vi "Begin.vi"(8 "error in":errorcluster) -> (0 "error out":errorcluster)   [LabVIEW 2019]
doc: "Called before other user functions, this VI is expected to open initial I/O refnums, load in file data, and do all program initialization. Notice that the <B>error out</B> terminal is simply used for data flow. Wiring it to other structures or subVIs ensures that this VI runs first."
uses:
  <vilib>/Rock Robotics/WPI/DriverStation/WPI_DriverStationRobotMode2.ctl
  <vilib>/Rock Robotics/WPI/Joystick/WPI_JoystickDeviceEnum.ctl
  <vilib>/Rock Robotics/WPI/ThirdParty/Phoenix-LabVIEW/Motor Controller/Controls/CTRE_Phoenix_MotorControl_NeutralMode.ctl
  Robot Global Data.vi
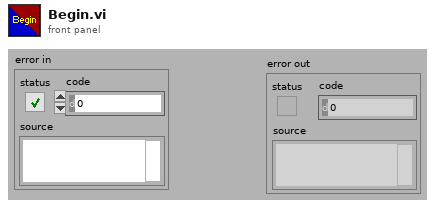
[diagram p1: front panel]
types:
  T1 = typedef "CTRE_Phoenix_MotorControl_NeutralMode.ctl" = enum8{"EEPROMSetting", "Override to Coast", "Override to Brake"}
  T2 = typedef "WPI_JoystickDeviceEnum.ctl" = enum16{"USB 0", "USB 1", "USB 2", "USB 3", "USB 4", "USB 5"}
  T3 = typedef "WPI_DriverStationRobotMode2.ctl" = enum16{"Autonomous Disabled", "Autonomous Enabled", "Teleop Disabled", "Teleop Enabled", "Disconnected", "Finish", "Test Disabled", "Test Enabled", "Emergency Stopped"}
  T4 = typedef "WPI_JoystickDevRef.ctl" = cluster{"Device":T2}
  T5 = typedef "WPI_MotorControlDeviceRef.ctl" = cluster{"DeviceStatus":errorcluster, "Type":T6, "PWM":cluster{"PWM Channel":T7, "DeadBand":T8}, "CAN":cluster{"Device Number":u8, "SetOutput VI Ref":variant, "GetOutput VI Ref":variant, "Enable VI Ref":variant, "Disable VI Ref":variant, "Data":variant}, "Invert":bool, "DIO PWM":cluster{"PWM \"Enable\" Channel":T7, "DIOChannel":T9, "PWM Rate":dbl}}
  T6 = typedef "WPI_MotorControlType.ctl" = enum16{"PWM", "CAN", "DIO PWM"}
  T7 = typedef "FPGA_DIOPWMChannel.ctl" = enum8{"PWM 0", "PWM 1", "PWM 2", "PWM 3", "PWM 4", "PWM 5", "PWM 6", "PWM 7", "PWM 8", "PWM 9", "PWM MXP 0", "PWM MXP 1", "PWM MXP 2", "PWM MXP 3", "PWM MXP 4", "PWM MXP 5", "PWM MXP 6", "PWM MXP 7", "PWM MXP 8", "PWM MXP 9", "Invalid"}
  T8 = typedef "WPI_PWMDeadband.ctl" = cluster{"Name":string, "maxPositivePwm":i32, "minPositivePwm":i32, "centerPwm":i32, "maxNegativePwm":i32, "minNegativePwm":i32, "angularRange":u16}
  T9 = typedef "FPGA_DIOChannel.ctl" = enum8{"DIO 0", "DIO 1", "DIO 2", "DIO 3", "DIO 4", "DIO 5", "DIO 6", "DIO 7", "DIO 8", "DIO 9", "DIO MXP 0", "DIO MXP 1", "DIO MXP 2", "DIO MXP 3", "DIO MXP 4", "DIO MXP 5", "DIO MXP 6", "DIO MXP 7", "DIO MXP 8", "DIO MXP 9", "DIO MXP 10", "DIO MXP 11", "DIO MXP 12", "DIO MXP 13", "DIO MXP 14", "DIO MXP 15", "SPI Port CS1", "SPI Port CS2", "SPI Port CS3", "SPI Port MISO", "SPI Port MOSI", "Invalid"}
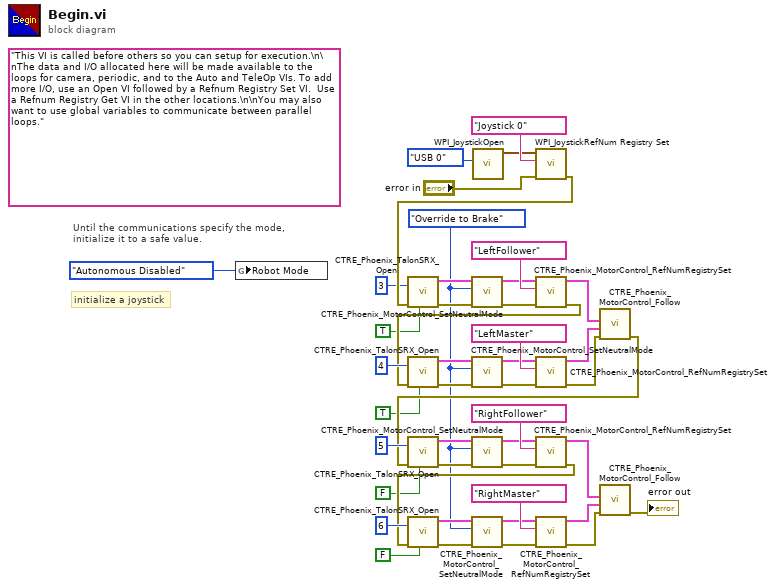
[diagram p0: block diagram]
diagram:
  w5 = CTRE_Phoenix_MotorControl_NeutralMode."Override to Brake" ("Motor Control Neutral Mode")
  (unwired) "This VI is called before others so you can setup for execution.\n\nThe data and I/O allocated here will be made available to the loops for camera, periodic, and to the Auto and TeleOp VIs. To add more I/O, use an Open VI followed by a Refnum Registry Set VI.  Use a Refnum Registry Get VI in the other locations.\n\nYou may also want to use global variables to communicate between parallel loops."
  # "initialize a joystick"
  # "Until the communications specify the mode,\ninitialize it to a safe value."
  n1 = global write "Robot Global Data.vi" "Robot Mode"(WPI_DriverStationRobotMode2."Autonomous Disabled" ("Robot Mode")) -> ()
  n2 = call <vilib>:"WPI_JoystickOpen.vi"("JoystickDevice"=WPI_JoystickDeviceEnum."USB 0") -> ("JoystickDevRef"=w43:T4)  [unwired: 10 in]
  n3 = call <vilib>:"WPI_JoystickRefNum Registry Set.vi"("error in (no error)"="error in", "refnum name"="Joystick 0", "JoystickDevRef"=w43) -> ("error out"=w41:errorcluster)  [unwired: 7 in, 1 out]
  n4 = call <vilib>:"CTRE_Phoenix_TalonSRX_Open.vi"("Invert"=TRUE, "error in"=w41, "Device Number"=u8 3) -> ("error out"=w24:errorcluster, "CAN Talon SRX Ref"=w25:T5)  [unwired: 7 in]
  n5 = call <vilib>:"CTRE_Phoenix_MotorControl_SetNeutralMode.vi"("error in (no error)"=w24, "Motor Control Neutral Mode"=w5, "PhoenixMotorControlDevRef"=w25) -> ("error out"=w23:errorcluster, "PhoenixMotorControlDevRef"=w4:T5)  [unwired: 7 in]
  n6 = call <vilib>:"CTRE_Phoenix_MotorControl_RefNumRegistrySet.vi"("error in (no error)"=w23, "refnum name"="LeftFollower", "PhoenixMotorControlDevRef"=w4) -> ("error out"=w10:errorcluster, "PhoenixMotorControlDevRef"=w30:T5)  [unwired: 7 in]
  n7 = call <vilib>:"CTRE_Phoenix_TalonSRX_Open.vi"("Invert"=TRUE, "error in"=w10, "Device Number"=u8 4) -> ("error out"=w21:errorcluster, "CAN Talon SRX Ref"=w22:T5)  [unwired: 7 in]
  n8 = call <vilib>:"CTRE_Phoenix_MotorControl_SetNeutralMode.vi"("error in (no error)"=w21, "Motor Control Neutral Mode"=w5, "PhoenixMotorControlDevRef"=w22) -> ("error out"=w19:errorcluster, "PhoenixMotorControlDevRef"=w20:T5)  [unwired: 7 in]
  n9 = call <vilib>:"CTRE_Phoenix_MotorControl_RefNumRegistrySet.vi"("error in (no error)"=w19, "refnum name"="LeftMaster", "PhoenixMotorControlDevRef"=w20) -> ("error out"=w9:errorcluster, "PhoenixMotorControlDevRef"=w29:T5)  [unwired: 7 in]
  n10 = call <vilib>:"CTRE_Phoenix_MotorControl_Follow.vi"("error in (no error)"=w9, "Master Controller to Follow"=w29, "PhoenixMotorControlDevRef"=w30) -> ("error out"=w8:errorcluster)  [unwired: 7 in, 1 out]
  n11 = call <vilib>:"CTRE_Phoenix_TalonSRX_Open.vi"("Invert"=FALSE, "error in"=w8, "Device Number"=u8 5) -> ("error out"=w17:errorcluster, "CAN Talon SRX Ref"=w18:T5)  [unwired: 7 in]
  n12 = call <vilib>:"CTRE_Phoenix_MotorControl_SetNeutralMode.vi"("error in (no error)"=w17, "Motor Control Neutral Mode"=w5, "PhoenixMotorControlDevRef"=w18) -> ("error out"=w15:errorcluster, "PhoenixMotorControlDevRef"=w16:T5)  [unwired: 7 in]
  n13 = call <vilib>:"CTRE_Phoenix_MotorControl_RefNumRegistrySet.vi"("error in (no error)"=w15, "refnum name"="RightFollower", "PhoenixMotorControlDevRef"=w16) -> ("error out"=w7:errorcluster, "PhoenixMotorControlDevRef"=w28:T5)  [unwired: 7 in]
  n14 = call <vilib>:"CTRE_Phoenix_TalonSRX_Open.vi"("Invert"=FALSE, "error in"=w7, "Device Number"=u8 6) -> ("error out"=w13:errorcluster, "CAN Talon SRX Ref"=w14:T5)  [unwired: 7 in]
  n15 = call <vilib>:"CTRE_Phoenix_MotorControl_SetNeutralMode.vi"("error in (no error)"=w13, "Motor Control Neutral Mode"=w5, "PhoenixMotorControlDevRef"=w14) -> ("error out"=w11:errorcluster, "PhoenixMotorControlDevRef"=w12:T5)  [unwired: 7 in]
  n16 = call <vilib>:"CTRE_Phoenix_MotorControl_RefNumRegistrySet.vi"("error in (no error)"=w11, "refnum name"="RightMaster", "PhoenixMotorControlDevRef"=w12) -> ("error out"=w6:errorcluster, "PhoenixMotorControlDevRef"=w27:T5)  [unwired: 7 in]
  n17 = call <vilib>:"CTRE_Phoenix_MotorControl_Follow.vi"("error in (no error)"=w6, "Master Controller to Follow"=w27, "PhoenixMotorControlDevRef"=w28) -> ("error out"=→"error out":errorcluster)  [unwired: 7 in, 1 out]
